vi "Intake_Execute.vi"() -> ()   [LabVIEW 2019]
uses:
  Utility_VIs/Basic_Motor_Modes.ctl
  Intake_Cluster.ctl
  Intake_States.ctl
  <vilib>/Rock Robotics/WPI/Solenoid/WPI_SolenoidValue.ctl
  Intake_Globals.vi
panel:
  in  "Intake_Speed":dbl=0.45
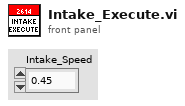
[diagram p1: front panel]
types:
  T1 = typedef "Basic_Motor_Modes.ctl" = enum16{"Percent_Voltage", "Speed_Control", "Position_Control", "Current"}
  T2 = typedef "Intake_Cluster.ctl" = cluster{"Control_State":T3, "Intake_On":bool, "Intake_Extended":bool, "Intake_Throttle":dbl, "Auto_Notifier":refnum<notifier>, "Parameter_1":dbl, "Parameter_2":dbl, "Step":dbl, "Outtake":bool}
  T3 = typedef "Intake_States.ctl" = enum16{"Manual_Throttle", "Manual_Single_Speed", "Compliant_Intake", "Command_RunIntake"}
  T4 = typedef "WPI_SolenoidValue.ctl" = enum16{"Off", "On", "Forward", "Reverse"}
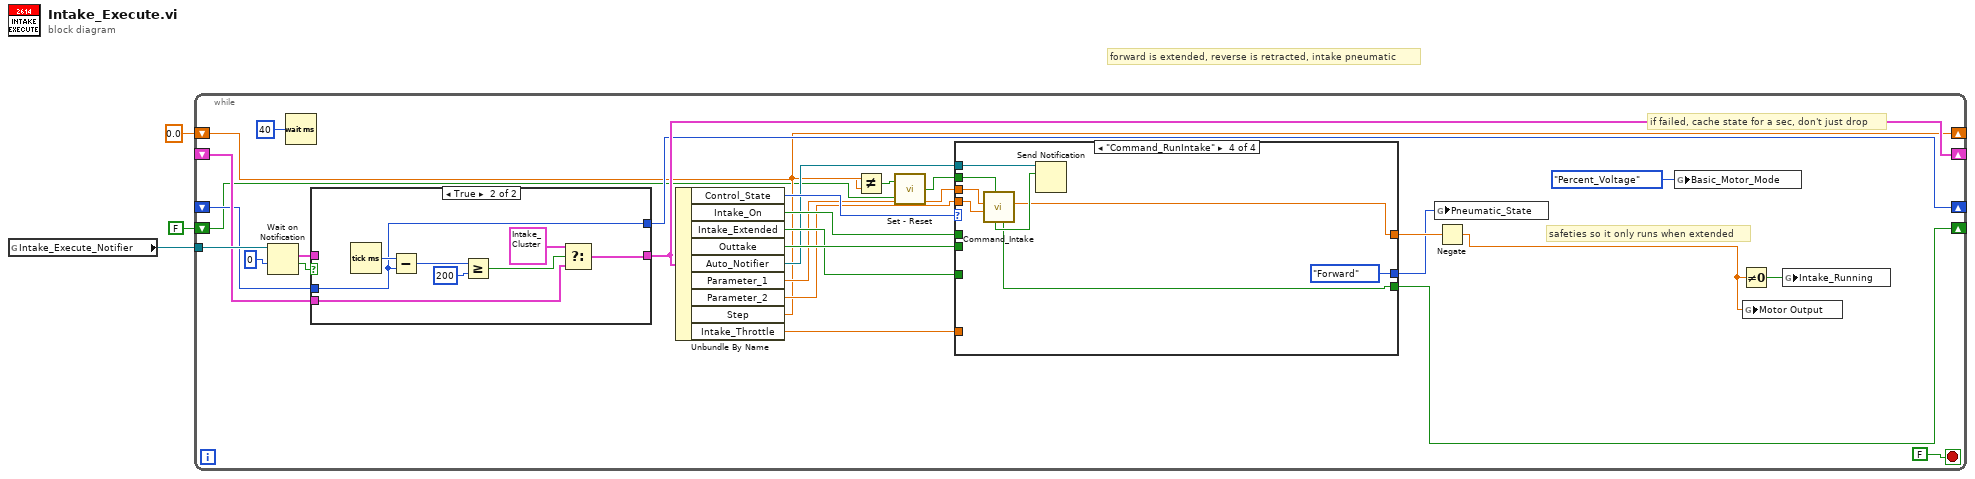
[diagram p0: block diagram]
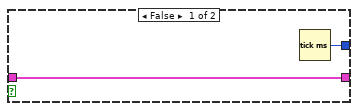
[diagram p2: hidden frame]
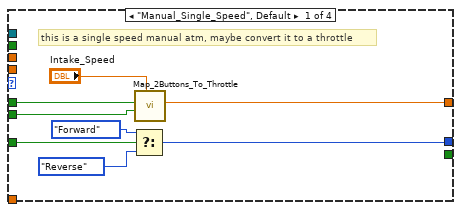
[diagram p3: hidden frame]
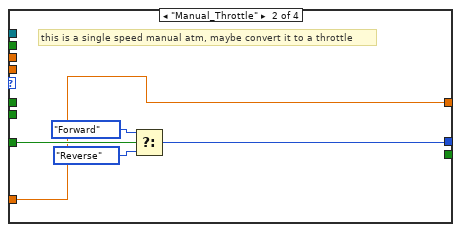
[diagram p4: hidden frame]
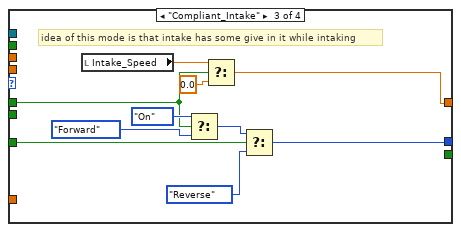
[diagram p5: hidden frame]
diagram:
  # "forward is extended, reverse is retracted, intake pneumatic"
  n1 = global read "Intake_Globals.vi" "Intake_Execute_Notifier"() -> (w3:refnum<notifier>)
  n2 = while {
    tunnel: w3 -> [w31]
    shift-right: [w20] -> _
    shift-left: _ -> [w19]
    shift-right: [w18] -> _
    shift-left: _ -> [w17]
    shift-right: [w13] -> _
    shift-left: 0.0 ("Step") -> [w12]
    shift-right: [w8] -> _
    shift-left: FALSE ("Reint") -> [w10]
    stop <- FALSE stop-if-true
    # "if failed, cache state for a sec, don't just drop"
    # "safeties so it only runs when extended"
    n3 = Wait on Notification(notifier=w31, timeout in ms (-1)=0) -> (notification=w21:T2, timed out?=w23:bool)  [unwired: 2 in, 2 out]
    n4 = Wait (ms)(milliseconds to wait=u32 40) -> ()  [unwired: 1 out]
    n5 = case shown="True" w23 {
      tunnel: w21 -> [w34 _]
      tunnel: [w34 w42] -> w20
      tunnel: w19 -> [_ w41]
      tunnel: [w33 w39] -> w18
      tunnel: w17 -> [_ w39]
      frame False {
        n6 = Tick Count (ms)() -> (millisecond timer value=w33:u32)
      }
      frame True {
        n7 = Tick Count (ms)() -> (millisecond timer value=w40:u32)
        n8 = Subtract(x=w40, y=w39) -> (x-y=w37:u32)
        n9 = Greater Or Equal?(x=w37, y=u32 200) -> (x >= y?=w38:bool)
        n10 = Select(t=T2 {"Control_State"=enum."Manual_Throttle", "Intake_On"=FALSE, "Intake_Extended"=FALSE, "Intake_Throttle"=0.0, "Auto_Notifier"=refnum, "Parameter_1"=0.0, "Parameter_2"=0.0, "Step"=0.0, "Outtake"=FALSE}, s=w38, f=w41) -> (s? t:f=w42:T2)
      }
    }
    n11 = Unbundle By Name(w20) -> ("Control_State"=w30:T3, "Intake_On"=w29:bool, "Intake_Extended"=w26:bool, "Outtake"=w27:bool, "Auto_Notifier"=w14:refnum<notifier>, "Parameter_1"=w16:dbl, "Parameter_2"=w15:dbl, "Step"=w13:dbl, "Intake_Throttle"=w5:dbl)
    n12 = Not Equal?(x=w13, y=w12) -> (x != y?=w11:bool)
    n13 = call "Set - Reset.vi"("Reset"=w10, "Set"=w11) -> ("Output"=w9:bool)
    n14 = case shown="\"Command_RunIntake\"" w30 {
      tunnel: w26 -> [w47 w52 w57 _]
      tunnel: [w48 w53 w62 WPI_SolenoidValue."Forward" ("Value")] -> w6
      tunnel: w29 -> [w46 _ w58 _]
      tunnel: [w43 w51 w56 w67] -> w25
      tunnel: w27 -> [w45 _ _ _]
      tunnel: w16 -> [_ _ _ w73]
      tunnel: w15 -> [_ _ _ w72]
      tunnel: w14 -> [_ _ _ w71]
      tunnel: w9 -> [_ _ _ w70]
      tunnel: [_ _ _ w68] -> w8
      tunnel: w5 -> [_ w51 _ _]
      frame "Manual_Single_Speed", Default {
        # "this is a single speed manual atm, maybe convert it to a throttle"
        n15 = Select(t=WPI_SolenoidValue."Forward" ("Value"), s=w47, f=WPI_SolenoidValue."Reverse" ("Value")) -> (s? t:f=w48:T4)
        n16 = call "Map_2Buttons_To_Throttle.vi"("Power"="Intake_Speed", "Down"=w45, "Up"=w46) -> ("Throttle"=w43:dbl)  [unwired: 8 in]
      }
      frame "Manual_Throttle" {
        # "this is a single speed manual atm, maybe convert it to a throttle"
        n17 = Select(t=WPI_SolenoidValue."Forward" ("Value"), s=w52, f=WPI_SolenoidValue."Reverse" ("Value")) -> (s? t:f=w53:T4)
      }
      frame "Compliant_Intake" {
        # "idea of this mode is that intake has some give in it while intaking"
        n18 = local read "Intake_Speed"() -> (w63:dbl)
        n19 = Select(t=WPI_SolenoidValue."On" ("Value"), s=w58, f=WPI_SolenoidValue."Forward" ("Value")) -> (s? t:f=w61:T4)
        n20 = Select(t=w63, s=w58, f=0.0) -> (s? t:f=w56:dbl)
        n21 = Select(t=w61, s=w57, f=WPI_SolenoidValue."Reverse" ("Value")) -> (s? t:f=w62:T4)
      }
      frame "Command_RunIntake" {
        n22 = call "Command_Intake.vi"("Startup"=w70, "Timeout"=w72, "Speed"=w73) -> ("Intake_Output"=w67:dbl, "Reint"=w68:bool, "Completed"=w69:bool)  [unwired: 6 in]
        n23 = Send Notification(notification=w69, notifier=w71) -> ()  [unwired: 1 in, 2 out]
      }
    }
    n24 = global write "Intake_Globals.vi" "Pneumatic_State"(w6) -> ()
    n25 = Negate(x=w25) -> (-x=w4:dbl)
    n26 = global write "Intake_Globals.vi" "Basic_Motor_Mode"(Basic_Motor_Modes."Percent_Voltage" ("Motor_Mode")) -> ()
    n27 = Not Equal To 0?(x=w4) -> (x != 0?=w24:bool)
    n28 = global write "Intake_Globals.vi" "Motor Output"(w4) -> ()
    n29 = global write "Intake_Globals.vi" "Intake_Running"(w24) -> ()
  }
